vi "Week_4_4.1_Ex-3.vi"() -> ()   [LabVIEW 2015]
panel:
  out "Waveform Graph":dynamicdata(graph)
  out "RMS":dbl format="%#_13g"
  out "Peak to Peak":dbl format="%#_13g"
  out "THD":dbl format="%#_13g"
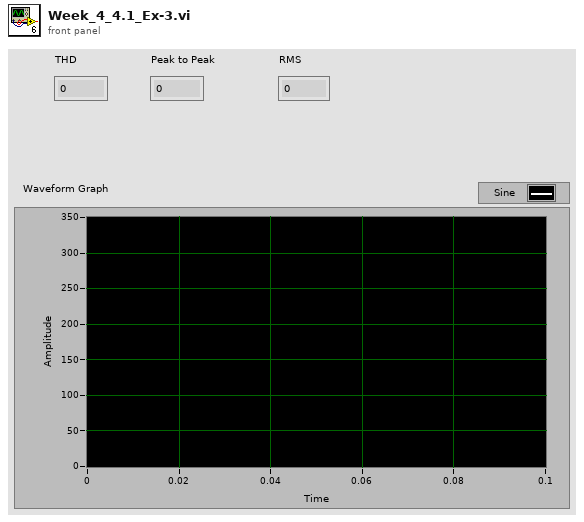
[diagram p1: front panel]
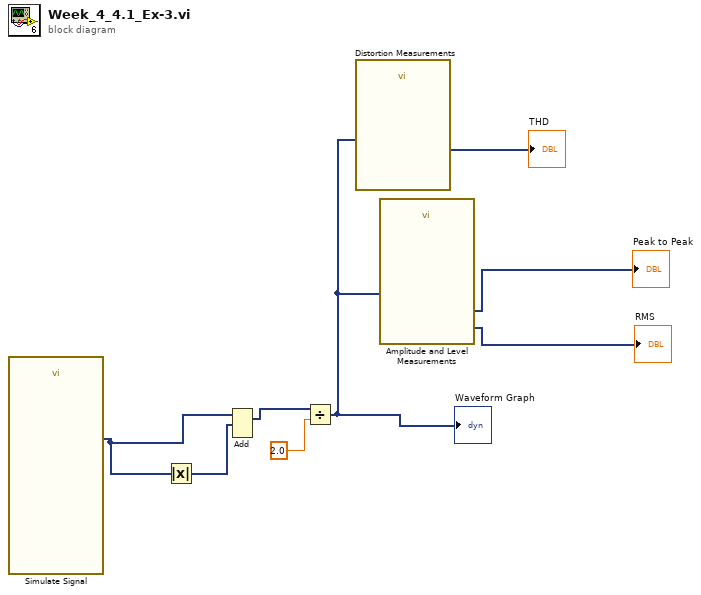
[diagram p0: block diagram]
diagram:
  n1 = call "Simulate Signal"() -> ("Sine"=w7:dynamicdata)  [unwired: 14 in, 1 out]
  n2 = Absolute Value(x=w7) -> (abs(x)=w6:dynamicdata)
  n3 = Add(1:w6, 2:w7) -> (0:w5:dynamicdata)  [unwired: 1 in, 1 out]
  n4 = Divide(x=w5, y=2.0) -> (x/y=w3:dynamicdata)
  "Waveform Graph" <- w3
  n5 = call "Distortion Measurements"("Signals"=w3) -> ("THD"=→"THD":dynamicdata)  [unwired: 8 in, 2 out]
  n6 = call "Amplitude and Level Measurements"("Signals"=w3) -> ("RMS"=→"RMS":dynamicdata, "Peak to Peak"=→"Peak to Peak":dynamicdata)  [unwired: 12 in, 1 out]
